vi "VISA_session_close.vi"(8 "error in (no error)":errorcluster, 11 "VISA resource name":refnum<visa-resource-name>) -> (0 "error out":errorcluster, 3 "VISA resource out":refnum<visa-resource-name>)   [LabVIEW 2015]
panel:
  # "This is valid for both:\n19572 & 19052"
  # "Close port"
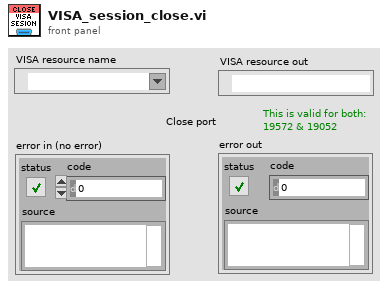
[diagram p1: front panel]
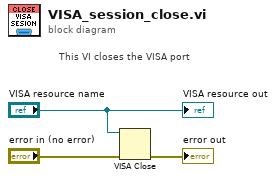
[diagram p0: block diagram]
diagram:
  # "This VI closes the VISA port"
  n1 = VISA Close(VISA resource name="VISA resource name", error in (no error)="error in (no error)") -> (error out=→"error out":errorcluster)
  "VISA resource out" <- "VISA resource name"
